vi "Get Result as Time.vi"(8 "error in (no error)":errorcluster, 10 "Use milliseconds":bool, 11 "Parameter in":refnum<class "Parameter.lvclass">) -> (0 "error out":errorcluster, 2 "Result":timestamp format="%<%.3X>T", 3 "Parameter out":refnum<class "Parameter.lvclass">)   [LabVIEW 2023, in "HAF.lvlib" / "Parameter.lvclass"]
doc: "Returns the Raw Result as a time only Timestamp with date defaulting to 01/01/1904. If Raw Result is not compatible then an error is raised."
uses:
  Parameter.lvclass
  Parameter.lvclass/Parameter.ctl
  HAF.lvlib
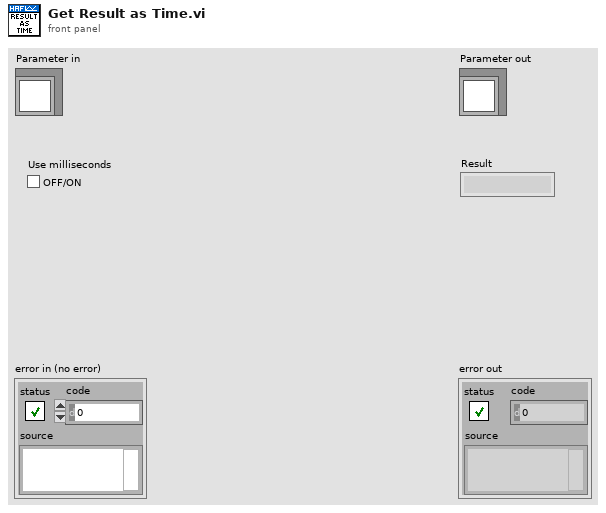
[diagram p1: front panel]
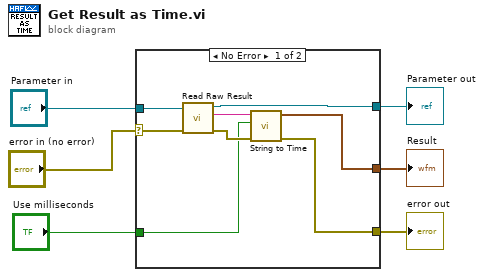
[diagram p0: block diagram]
diagram:
  n1 = case shown="No Error" "error in (no error)" {
    selector: "error in (no error)" -> [w13 w16]
    tunnel: [w8 w16] -> w5
    tunnel: [w10 w15] -> w3
    tunnel: "Parameter in" -> [w14 w15]
    tunnel: [w9 _] -> w2
    tunnel: "Use milliseconds" -> [w7 _]
    frame No Error {
      n2 = call-dynamic "Read Raw Result.vi"("error in (no error)"=w13, "Parameter in"=w14) -> ("error out"=w11:errorcluster, "Raw Result"=w12:string, "Parameter out"=w10:refnum<class "Parameter.lvclass">)  [unwired: 7 in]
      n3 = call "String to Time.vi"("error in (no error)"=w11, "Include ms"=w7, "String to Convert"=w12) -> ("error out"=w8:errorcluster, "Time Value"=w9:timestamp)  [unwired: 7 in]
    }
    frame Error {
    }
  }
  "error out" <- w5
  "Parameter out" <- w3
  "Result" <- w2
